vi "Initialize.vi"(8 "error in (no error)":errorcluster, 10 "Parser Name":string, 11 "STDF File Parser in":refnum<class "STDF File Parser.lvclass">) -> (0 "error out":errorcluster, 3 "STDF File Parser out":refnum<class "STDF File Parser.lvclass">)   [LabVIEW 2018, in "STDF File Parser.lvclass"]
uses:
  STDF File Parser.lvclass
  STDF File Parser.lvclass/STDF File Parser.ctl
  TestDataMgr/TestDataMgr.lvclass
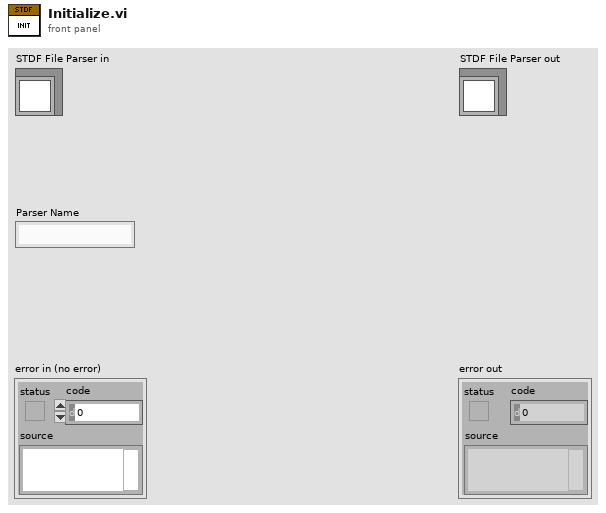
[diagram p1: front panel]
types:
  T1 = typedef "TestDataMgr.lvclass/Session Handle.ctl" = refnum<data-value>
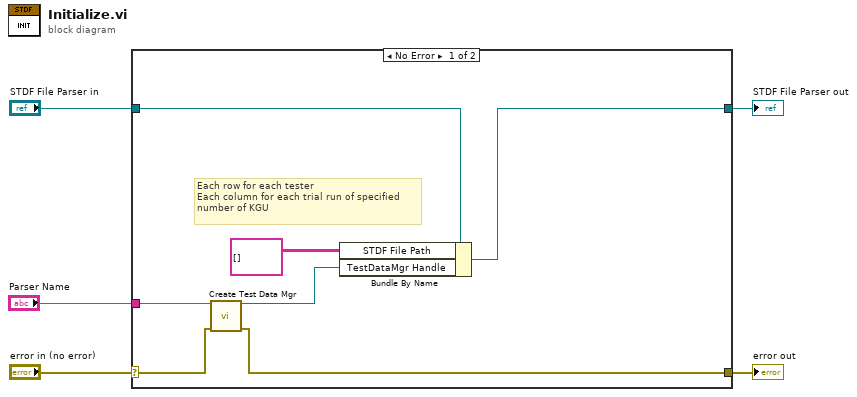
[diagram p0: block diagram]
diagram:
  n1 = case shown="No Error" "error in (no error)" {
    selector: "error in (no error)" -> [w11 w14]
    tunnel: [w10 w14] -> w4
    tunnel: [w6 w13] -> w2
    tunnel: "STDF File Parser in" -> [w9 w13]
    tunnel: "Parser Name" -> [w12 _]
    frame No Error {
      # "Each row for each tester\nEach column for each trial run of specified\nnumber of KGU"
      n2 = call "Create Test Data Mgr.vi"("Session  Name ()"=w12, "error in (no error)"=w11) -> ("Session Handle"=w7:T1, "error out"=w10:errorcluster)  [unwired: 12 in]
      n3 = Bundle By Name(cluster=w9, "STDF File Path"=string[][] [] ("STDF Files"), "TestDataMgr Handle"=w7) -> (w6:refnum<class "STDF File Parser.lvclass">)
    }
    frame Error {
    }
  }
  "error out" <- w4
  "STDF File Parser out" <- w2
